vi "PH_Sequencer.set GUI elements to default.vi"(0 "i ref in":refnum<vi>, 5 "error in (no error)":errorcluster) -> (14 "i ref out":refnum<vi>, 19 "error out":errorcluster)   [LabVIEW 2014, in "PH_Sequencer.lvlib"]
doc: "This VI sets some GUI elements to dafault (start) values."
uses:
  PH_Sequencer.lvlib
  PH_Basics/PH_PP_Common/PH_PP_Common.PUs.ctl
  PH_Basics/PH_Common/PH_Common.lvlib
  PH_BeamlineInformation/PH_BeamlineInformation.lvlib
  PH_Basics/PH_PP_Common/PH_PP_Common.lvlib
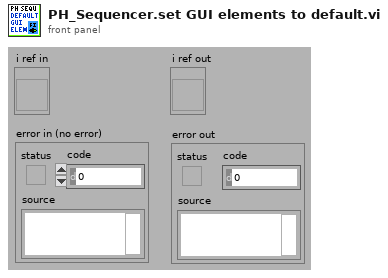
[diagram p1: front panel]
types:
  T1 = typedef "PH_PP_Common.lvlib/PH_PP_Common.PUs.ctl" = enum16{"no Info", "PA-19mm-1", "PA-19mm-2", "PA-45mm-PILC", "PA-45mm-MAIN", "MA-PU-1", "MA-PU-2", "MA-PU-3", "MA-PU-4", "MA-PU-5", "MA-PU-6", "MA-FR", "MA-PILC", "PA-45mm-DP"}
  T2 = typedef "PH_Sequencer.lvlib/PH_Sequencer.i attribute.ctl" = cluster{"GUI Refs":cluster{"Main Off":refnum<vi>, "Fire":refnum<vi>, "Status":refnum<vi>, "Ready":refnum<vi>, "Waiting Time":refnum<vi>, "Timeout":refnum<vi>, "PPMA Ready":refnum<vi>, "Sequencer SM State":refnum<vi>, "PPPA Ready":refnum<vi>, "Calorimeter":refnum<vi>, "Beamline Ready":refnum<vi>, "Clear Beamline":refnum<vi>, "Linkage PPMA Rods":refnum<vi>, "Linkage Current PA":refnum<vi>, "Linkage Current MA":refnum<vi>, "Timing Ready":refnum<vi>, "State Timing":refnum<vi>, "Force Timing":refnum<vi>, "PSDB Shot Comment":refnum<vi>, "State PA Backreflection":refnum<vi>, "Beamline Z6 Ready":refnum<vi>, "Clear Z6 Beamline":refnum<vi>, "Sequence length":refnum<vi>, "Timing Mode":refnum<vi>, "Slow Trigger Settings":refnum<vi>, "Experiment Description":refnum<vi>, "State PSDB":refnum<vi>, "PSDB Ready":refnum<vi>, "Set PSDB Settings":refnum<vi>, "Get PSDB Info":refnum<vi>, "Take Snapshot":refnum<vi>, "Shottype":refnum<vi>, "Experiment":refnum<vi>, "Phase Frontends":refnum<vi>, "PP 45mm PILC in use":refnum<vi>}, "Status Info":cluster{"Machine Status":T3, "WaitingTime":i32, "Timeout":bool}, "Readyness":cluster{"Ready to shot":bool, "PPMA Ready":bool, "PPPA Ready":bool, "BL Ready":bool, "Timing Ready":bool, "BL Z6 Ready":bool, "PSDBReady":bool}, "Instancenames":cluster{"PPMA Rods":string, "PP Current Meas":string, "PH Beamline Chief":string, "PA Backrefl Meas":string, "Z6 Beamline Chief":string}, "Data to read":bool, "Calorimeter":cluster{"Instancename":string, "On":bool, "linked":bool}, "Linkage":cluster{"PPMA Rods":bool, "PP Current Meas":bool, "PHELIX Beamline Chief":bool, "PA Backrefl Meas":bool, "Z6 Beamline Chief":bool}, "Timing":cluster{"Instance":string, "linked":bool, "Status":T3, "Timing Mode":T4, "Slow Trigger Settings":T5, "Info available":cluster{"ext SlowTrigger":bool, "T2":bool, "Mode":bool, "Delay Slow Trigger":bool, "Phase FEs":bool}, "FE Phase":T6}, "Service ID R2S":i32, "PSDB":cluster{"Controller Instance":string, "Controller Status":T3, "Controller linked":bool, "Settings acknowledged":bool, "Current Experiment ID":i16, "Current Shot Type":i16, "Current Comment":string, "Remember Settings":bool, "Write 2 early":bool}, "PSDB Data":cluster{"Main Off?":bool, "Sequence Length":dbl, "Sequence startet":timestamp}, "6P 4Q Positions":cluster{"Instancename":string, "linked":bool, "Position":T7}[], "PUs":T8[]}
  T3 = typedef "PH_StatusHandler.lvlib/PH_StatusHandler.Status.ctl" = i16
  T4 = typedef "PH_Timing.lvlib/PH_Timing.Timing Mode.ctl" = cluster{"T2":i16, "Modeselector":enum32{"10 Hz", "0.5 Hz", "Shot"}}
  T5 = typedef "PH_Timing.lvlib/PH_Timing.Slow Trigger Settings.ctl" = cluster{"Delay":dbl, "externally triggered?":bool}
  T6 = typedef "PH_Timing.lvlib/PH_Timing.Phase FEs.ctl" = cluster{"Phase":dbl}
  T7 = typedef "PH_4_Pos_Selector.lvlib/PH_4_Pos_Selector.Position Selector.ctl" = u16
  T8 = typedef "PH_Sequencer.lvlib/PH_Sequencer.Head.ctl" = cluster{"PowerUnit":T1, "GUI Ref":refnum<vi>, "Information":T9, "linked?":bool, "GUI Ref Current Voltage":refnum<vi>}
  T9 = typedef "PH_Sequencer.lvlib/PH_Sequencer.PU Information.ctl" = cluster{"State":T3, "Waiting Time [s]":dbl, "PU State SM":T10, "PU Timeout SM":T10}
  T10 = typedef "PH_PowerUnit_BaseClass.lvlib/PH_PowerUnit_BaseClass.SM States.ctl" = enum16{".", "Stand by", "Switch PU on", "Configure", "Set Default Voltage", "Set STANDBY", "Set READY", "Wait for Shot Cmd", "Open Dump Rods", "Open Ross Relais", "Close Ross Relais", "Switch PSU on", "Switch PSU off", "Charge", "Switch GD Channel on", "Close Dump Rods", "Rods-TO", "RR-TO", "PSU-TO", "Trigger-TO"}
  T11 = typedef "PH_BeamlineInformation.lvlib/PH_BeamlineInformation.i attribute.ctl" = cluster{"BL GUI Elements of Services":cluster{"Service Name":string, "GUI Elements":refnum<vi>[], "Status":i32}[], "Powermeters":T12, "Efficiency":T13, "Heads":T14[]}
  T12 = typedef "PH_BeamlineInformation.lvlib/PH_BeamlineInformation.Powermeter.ctl" = cluster{"ns FE":cluster{"GUI Ref":refnum<vi>, "Value":dbl}, "fs FE":cluster{"GUI Ref":refnum<vi>, "Value":dbl}, "PA":cluster{"GUI Ref":refnum<vi>, "Value":dbl}, "MA":cluster{"GUI Ref":refnum<vi>, "Value":dbl}, "Z6 green":cluster{"GUI Ref":refnum<vi>, "Value":dbl}, "Z6 IR":cluster{"GUI Ref":refnum<vi>, "Value":dbl}, "Z6 COS":cluster{"GUI Ref":refnum<vi>, "Value":dbl}}
  T13 = typedef "PH_BeamlineInformation.lvlib/PH_BeamlineInformation.Efficiency.ctl" = cluster{"PA Gain":cluster{"GUI Ref":refnum<vi>, "Value":dbl}, "MA Gain":cluster{"GUI Ref":refnum<vi>, "Value":dbl}, "Z6 green Conversion":cluster{"GUI Ref":refnum<vi>, "Value":dbl}, "Z6 Comp Losses":cluster{"GUI Ref":refnum<vi>, "Value":dbl}}
  T14 = typedef "PH_BeamlineInformation.lvlib/PH_BeamlineInformation.Head.ctl" = cluster{"PowerUnit":T1, "in use":cluster{"Value":bool, "GUI Ref":refnum<vi>, "linked":bool}, "voltage":cluster{"Value":dbl, "GUI Ref":refnum<vi>, "linked":bool}}
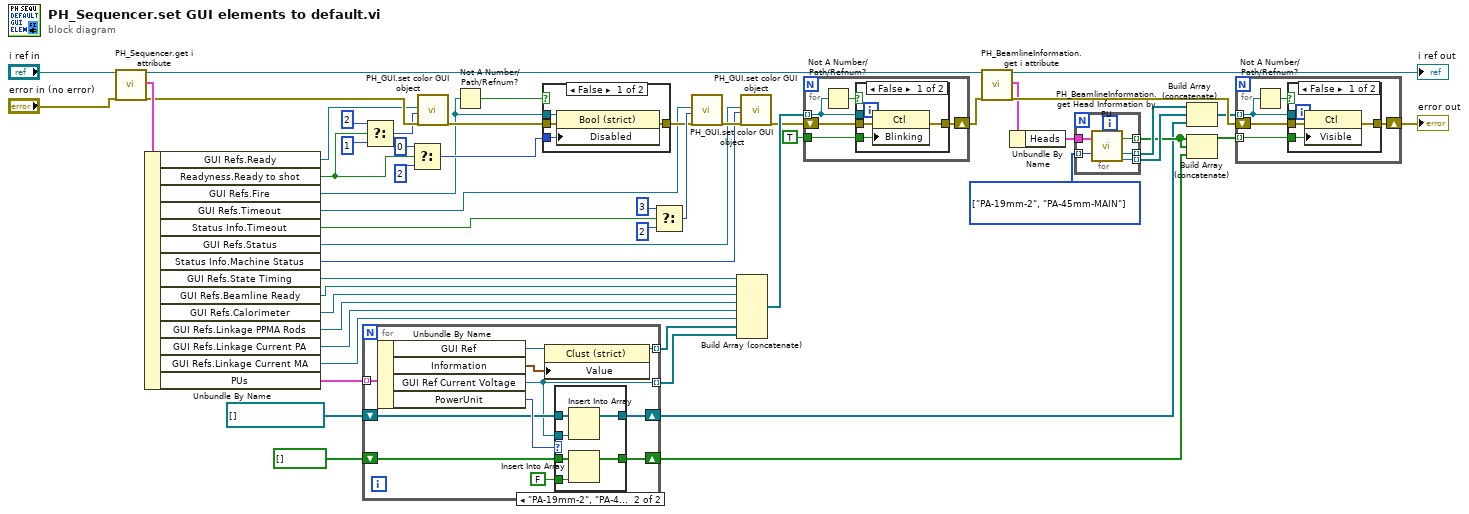
[diagram p0: block diagram]
diagram:
  w11 = T1[] [enum."PA-19mm-2", enum."PA-45mm-MAIN"] items=["no Info", "PA-19mm-1", "PA-19mm-2", "PA-45mm-PILC", "PA-45mm-MAIN", "MA-PU-1", "MA-PU-2", "MA-PU-3", "MA-PU-4", "MA-PU-5", "MA-PU-6", "MA-FR", "MA-PILC", "PA-45mm-DP"]
  n1 = call "PH_Sequencer.get i attribute.vi"("i ref in"="i ref in", "error in (no error)"="error in (no error)") -> ("i ref out"=w15:refnum<vi>, "i attribute"=w51:T2, "error out"=w44:errorcluster)  [unwired: 15 in]
  n2 = Unbundle By Name(w51) -> ("GUI Refs.Ready"=w36:refnum<vi>, "Readyness.Ready to shot"=w30:bool, "GUI Refs.Fire"=w28:refnum<vi>, "GUI Refs.Timeout"=w27:refnum<vi>, "Status Info.Timeout"=w41:bool, "GUI Refs.Status"=w25:refnum<vi>, "Status Info.Machine Status"=w24:T3, "GUI Refs.State Timing"=w48:refnum<vi>, "GUI Refs.Beamline Ready"=w47:refnum<vi>, "GUI Refs.Calorimeter"=w46:refnum<vi>, "GUI Refs.Linkage PPMA Rods"=w45:refnum<vi>, "GUI Refs.Linkage Current PA"=w23:refnum<vi>, "GUI Refs.Linkage Current MA"=w22:refnum<vi>, "PUs"=w20:T8[])
  n3 = for {
    tunnel: w20 -> [w63] mode=indexing
    tunnel: [w61] -> w19 mode=indexing
    tunnel: [w57] -> w5 mode=indexing
    shift-right: [w56] -> w2
    shift-left: refnum<vi>[] [] -> [w59]
    shift-right: [w55] -> w1
    shift-left: bool[] [] -> [w58]
    n4 = Unbundle By Name(w63) -> ("GUI Ref"=w64:refnum<vi>, "Information"=w62:T9, "GUI Ref Current Voltage"=w57:refnum<vi>, "PowerUnit"=w60:T1)
    n5 = property class="Clust (strict)"(reference=w64, "Value"=w62) -> (reference out=w61:refnum<vi>)  [unwired: 1 in, 1 out]
    n6 = case shown="\"PA-19mm-2\", \"PA-45mm-MAIN\"" w60 {
      tunnel: w57 -> [_ w72]
      tunnel: [w66 w71] -> w56
      tunnel: w59 -> [w66 w70]
      tunnel: FALSE -> [_ w69]
      tunnel: [w65 w68] -> w55
      tunnel: w58 -> [w65 w67]
      frame Default {
      }
      frame "PA-19mm-2", "PA-45mm-MAIN" {
        n7 = Insert Into Array(array=w70, new element=w72) -> (w71:refnum<vi>[])  [unwired: 1 in]
        n8 = Insert Into Array(array=w67, new element=w69) -> (w68:bool[])  [unwired: 1 in]
      }
    }
  }
  n9 = Select(t=2, s=w30, f=1) -> (s? t:f=w37:i32)
  n10 = Select(t=0, s=w30, f=2) -> (s? t:f=w29:i32)
  n11 = call "PH_GUI.set color GUI object.vi"("GUI object Ref"=w36, "State"=w37, "error in (no error)"=w44) -> ("error out"=w34:errorcluster)  [unwired: 16 in]
  n12 = Not A Number/Path/Refnum?(number/path/refnum=w28) -> (NaN/Path/Refnum?=w35:bool)
  n13 = case shown="False" w35 {
    tunnel: w28 -> [w76 _]
    tunnel: w34 -> [w75 w77]
    tunnel: [w74 w77] -> w33
    tunnel: w29 -> [w73 _]
    frame False {
      n14 = property class="Bool (strict)"(reference=w76, error in=w75, "Disabled"=w73) -> (error out=w74:errorcluster)  [unwired: 1 out]
    }
    frame True {
    }
  }
  n15 = Select(t=3, s=w41, f=2) -> (s? t:f=w40:i32)
  n16 = call "PH_GUI.set color GUI object.vi"("GUI object Ref"=w27, "State"=w40, "error in (no error)"=w33) -> ("error out"=w26:errorcluster)  [unwired: 16 in]
  n17 = Build Array (concatenate)(w48, w47, w46, w45, w23, w22, w19, w5) -> (w50:refnum<vi>[])
  n18 = call "PH_GUI.set color GUI object.vi"("GUI object Ref"=w25, "State"=w24, "error in (no error)"=w26) -> ("error out"=w21:errorcluster)  [unwired: 16 in]
  n19 = for {
    tunnel: w50 -> [w79] mode=indexing
    tunnel: TRUE -> [w82]
    shift-right: [w81] -> w18
    shift-left: w21 -> [w80]
    n20 = Not A Number/Path/Refnum?(number/path/refnum=w79) -> (NaN/Path/Refnum?=w78:bool)
    n21 = case shown="False" w78 {
      tunnel: w79 -> [w86 _]
      tunnel: w82 -> [w85 _]
      tunnel: [w84 w87] -> w81
      tunnel: w80 -> [w83 w87]
      frame False {
        n22 = property class="Ctl"(reference=w86, error in=w83, "Blinking"=w85) -> (error out=w84:errorcluster)  [unwired: 1 out]
      }
      frame True {
      }
    }
  }
  n23 = call "PH_BeamlineInformation.get i attribute.vi"("i ref in"=w15, "error in (no error)"=w18) -> ("i ref out"=→"i ref out":refnum<vi>, "i attribute"=w13:T11, "error out"=w16:errorcluster)  [unwired: 15 in]
  n24 = Unbundle By Name(w13) -> ("Heads"=w12:T14[])
  n25 = for {
    tunnel: w12 -> [w92]
    tunnel: w11 -> [w91] mode=indexing
    tunnel: [w89] -> w6 mode=indexing
    tunnel: [w90] -> w10 mode=indexing
    tunnel: [w88] -> w7 mode=indexing
    n26 = call "PH_BeamlineInformation.get Head Information by PU.vi"("Heads"=w92, "Power Unit"=w91) -> ("In Use linked?"=w89:bool, "In Use GUI Ref"=w90:refnum<vi>, "Voltage GUI Ref"=w88:refnum<vi>)  [unwired: 12 in, 3 out]
  }
  n27 = Build Array (concatenate)(w10, w7, w2) -> (w9:refnum<vi>[])
  n28 = Build Array (concatenate)(w6, w6, w1) -> (w8:bool[])
  n29 = for {
    tunnel: w9 -> [w94] mode=indexing
    tunnel: w8 -> [w97] mode=indexing
    shift-right: [w96] -> w17
    shift-left: w16 -> [w95]
    n30 = Not A Number/Path/Refnum?(number/path/refnum=w94) -> (NaN/Path/Refnum?=w93:bool)
    n31 = case shown="False" w93 {
      tunnel: w94 -> [w101 _]
      tunnel: w97 -> [w100 _]
      tunnel: [w99 w102] -> w96
      tunnel: w95 -> [w98 w102]
      frame False {
        n32 = property class="Ctl"(reference=w101, error in=w98, "Visible"=w100) -> (error out=w99:errorcluster)  [unwired: 1 out]
      }
      frame True {
      }
    }
  }
  "error out" <- w17
